vi "Find Control Ref with KeyFocused.vi"(8 "错误输入（无错误）":errorcluster, 11 "VI Ref":refnum<vi>) -> (0 "错误输出":errorcluster, 1 "控件已找到？":bool, 3 "查找带键选中的控件":refnum<vi>)   [LabVIEW 2012]
uses:
  VIRef.lvlib
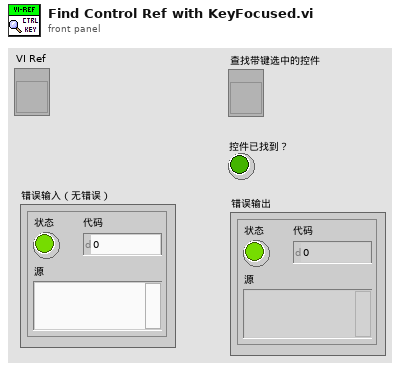
[diagram p1: front panel]
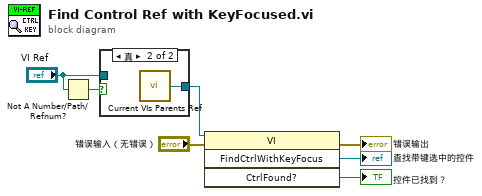
[diagram p0: block diagram]
diagram:
  n1 = Not A Number/Path/Refnum?(number/path/refnum="VI Ref") -> (NaN/Path/Refnum?=w7:bool)
  n2 = case shown="真" w7 {
    tunnel: [w8 w9] -> w5
    tunnel: "VI Ref" -> [w8 _]
    frame False {
    }
    frame True {
      n3 = call "Current VIs Parents Ref.vi"() -> ("Calling VI's Reference"=w9:refnum<vi>)  [unwired: 2 in]
    }
  }
  n4 = invoke class="VI" method="FindCtrlWithKeyFocus"(reference=w5, error in="错误输入（无错误）") -> (error out=→"错误输出":errorcluster, "FindCtrlWithKeyFocus"=→"查找带键选中的控件":refnum<vi>, "CtrlFound?"=→"控件已找到？":bool)  [unwired: 2 in, 1 out]
